vi "Layers To Decorate.vi"(9 "Actor To Decorate":refnum<class "Actor.lvclass">, 10 "Layers":refnum<class "Actor.lvclass">[](array[class])) -> (2 "Decorated Actor":refnum<class "Actor.lvclass">)   [LabVIEW 2025, in "jettl.lvlib"]
uses:
  jettl.lvlib
  Actor/Actor.lvclass
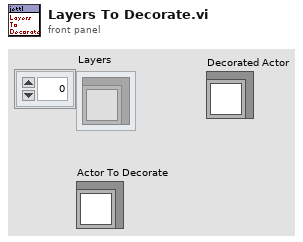
[diagram p1: front panel]
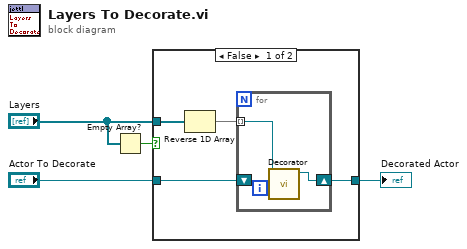
[diagram p0: block diagram]
diagram:
  n1 = Empty Array?(array="Layers") -> (empty?=w1:bool)
  n2 = case shown="False" w1 {
    tunnel: "Actor To Decorate" -> [w7 w12]
    tunnel: [w6 w12] -> w3
    tunnel: "Layers" -> [w5 _]
    frame False {
      n3 = Reverse 1D Array(array=w5) -> (reversed array=w8:refnum<class "Actor.lvclass">[])
      n4 = for {
        tunnel: w8 -> [w10] mode=indexing
        shift-right: [w9] -> w6
        shift-left: w7 -> [w11]
        n5 = call-dynamic "Decorator.vi"("Actor"=w11, "Actor in"=w10) -> ("Actor out"=w9:refnum<class "Actor.lvclass">)  [unwired: 9 in]
      }
    }
    frame True {
    }
  }
  "Decorated Actor" <- w3
